vi "Fat A.vi"(11 "GIC Input":T1={"     Use ?\nOff       On"=[FALSE, TRUE, FALSE, TRUE], "Mode:"=FALSE, "Extra Port"="", "Hokuyo Port"="COM7", "Tx Prop  Port"="COM6", "Compass Port"="", "GPS Port"="", "Num of WPs"=0, "WP Lats and Longs"={"WP Lats"=[], "WP Longs"=[]}, "Obst Lats and Longs"={"Obst Lats"=[], "Obst Longs"=[]}, "Parameters"=[], "GPS Data"=[], "Compass"=0.0, "LMS Vector"=[], "Vision Vector"=[], "Direction Cmd"=0.0, "Speed Cmd"=0.0, "WP Vector"=[], "WP Number"=0, "Extra"=0, "SW Map"=[], "Path Cluster"={"Path x node"=[], "Path y node"=[]}, "Sim Course"=[]} {"Obst Lats and Longs"."Obst Longs" format="%#_8g"; "Obst Lats and Longs"."Obst Lats" format="%#_8g"}) -> (3 "GIC Output":T1={"     Use ?\nOff       On"=[FALSE, TRUE, FALSE, TRUE], "Mode:"=FALSE, "Extra Port"="", "Hokuyo Port"="COM7", "Tx Prop  Port"="COM6", "Compass Port"="", "GPS Port"="", "Num of WPs"=0, "WP Lats and Longs"={"WP Lats"=[], "WP Longs"=[]}, "Obst Lats and Longs"={"Obst Lats"=[], "Obst Longs"=[]}, "Parameters"=[], "GPS Data"=[], "Compass"=0.0, "LMS Vector"=[], "Vision Vector"=[], "Direction Cmd"=0.0, "Speed Cmd"=0.0, "WP Vector"=[], "WP Number"=0, "Extra"=0, "SW Map"=[], "Path Cluster"={"Path x node"=[], "Path y node"=[]}, "Sim Course"=[]} {"Obst Lats and Longs"."Obst Longs" format="%#_8g"; "Obst Lats and Longs"."Obst Lats" format="%#_8g"})   [LabVIEW 2014]
panel:
  out "Array":dbl[](array[numeric])
  out "Numeric":dbl
  out "Test SWMap Out":dbl[][](array[numeric])
  in  "Test Fat":dbl=1.0
  # "Fat A"
  # "Input:"
  # "Output:"
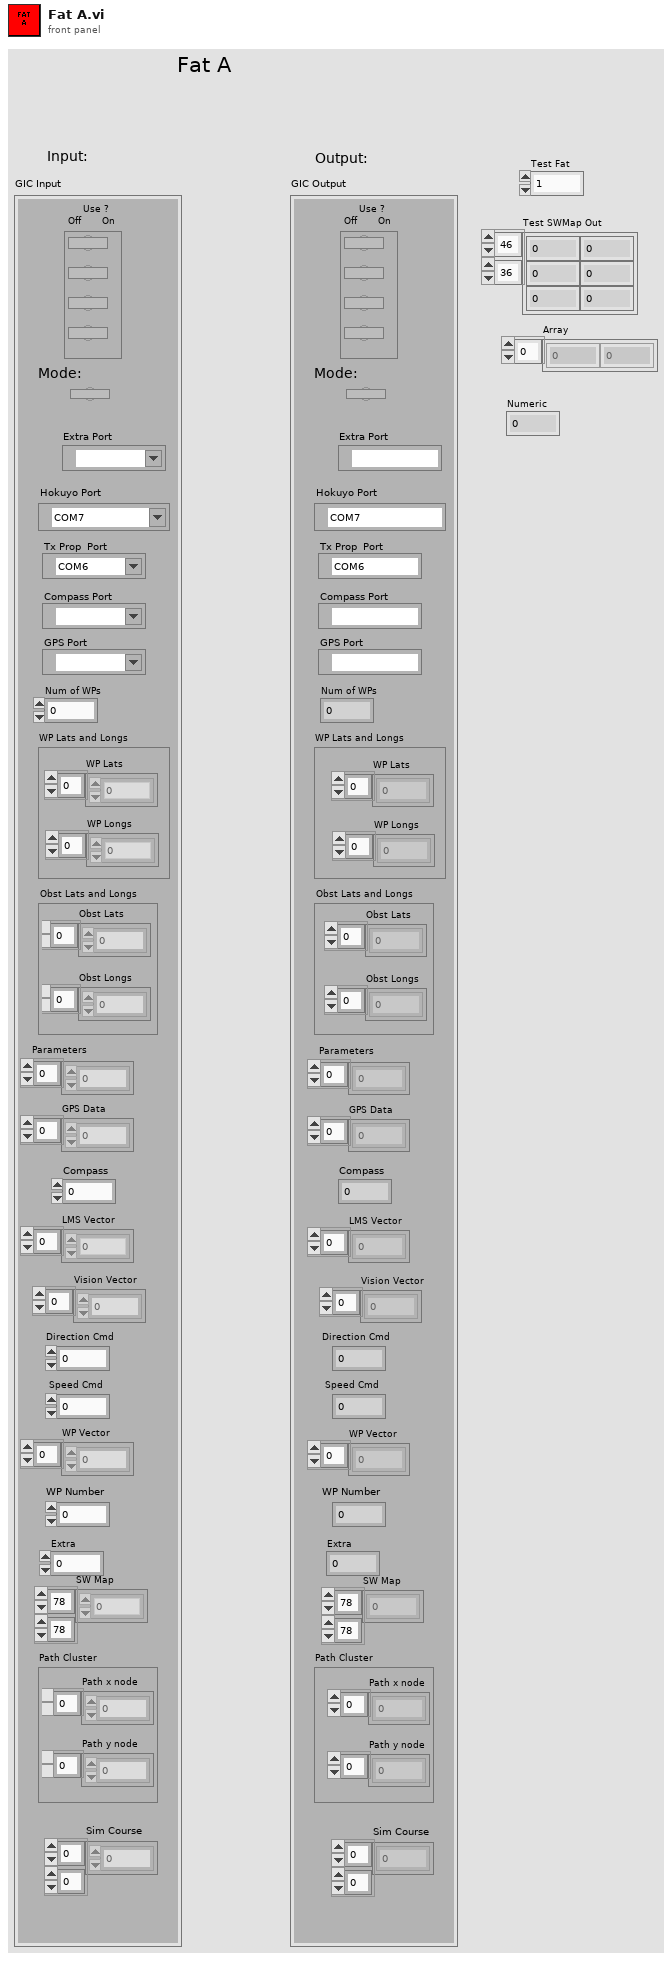
[diagram p1: front panel]
types:
  T1 = cluster{"     Use ?\nOff       On":bool[], "Mode:":bool, "Extra Port":refnum<visa-resource-name>, "Hokuyo Port":refnum<visa-resource-name>, "Tx Prop  Port":refnum<visa-resource-name>, "Compass Port":refnum<visa-resource-name>, "GPS Port":refnum<visa-resource-name>, "Num of WPs":i16, "WP Lats and Longs":cluster{"WP Lats":dbl[], "WP Longs":dbl[]}, "Obst Lats and Longs":cluster{"Obst Lats":dbl[], "Obst Longs":dbl[]}, "Parameters":dbl[], "GPS Data":dbl[], "Compass":dbl, "LMS Vector":dbl[], "Vision Vector":dbl[], "Direction Cmd":dbl, "Speed Cmd":dbl, "WP Vector":dbl[], "WP Number":i32, "Extra":i16, "SW Map":i32[][], "Path Cluster":cluster{"Path x node":dbl[], "Path y node":dbl[]}, "Sim Course":i8[][]}
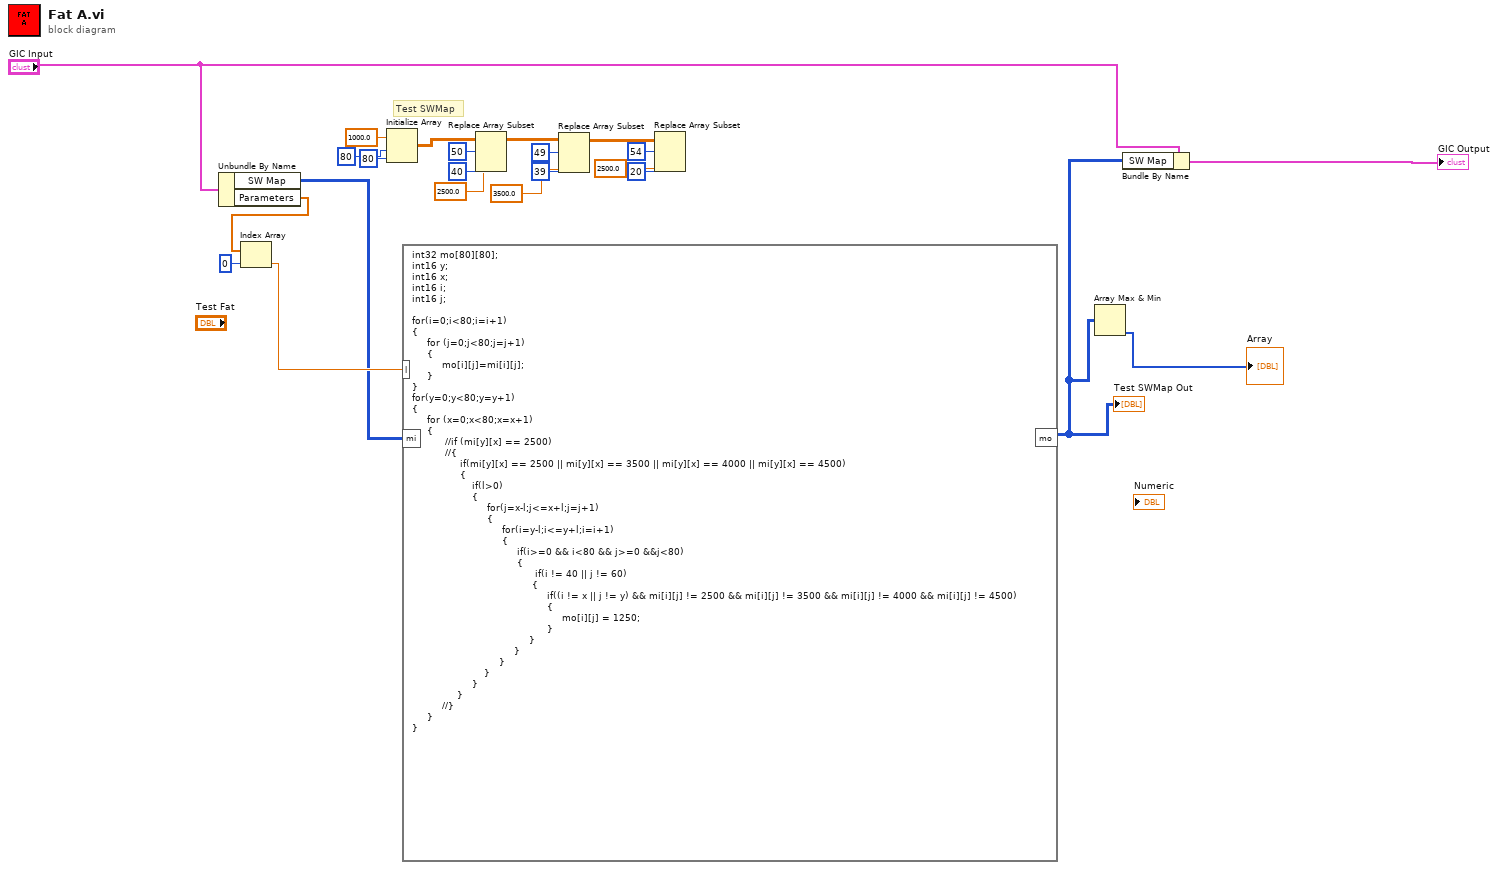
[diagram p0: block diagram]
diagram:
  # "Test SWMap"
  n1 = Unbundle By Name("GIC Input") -> ("SW Map"=w3:i32[][], "Parameters"=w12:dbl[])
  n2 = Index Array(array=w12, index=0) -> (element=w4:dbl)
  n3 = Initialize Array(1000.0 ("element"), 80 ("dimension size"), 80 ("dimension size")) -> (w20:dbl[][])
  n4 = formula code="int32 mo[80][80];\nint16 y;\nint16 x;\nint16 i;\nint16 j;\n\nfor(i=0;i<80;i=i+1)\n{\n     for (j=0;j<80;j=j+1)\n     {\n          mo[i][j]=mi[i][j];\n     }\n}\nfor(y=0;y<80;y=y+1)\n{\n     for (x=0;x<80;x=x+1)\n     {\n           //if (mi[y][x] == 2500)\n           //{\n                if(mi[y][x] == 2500 || mi[y][x] == 3500 || mi[y][x] == 4000 || mi[y][x] == 4500)\n                {\n                    if(l>0)\n                    {\n                         for(j=x-l;j<=x+l;j=j+1)\n                         {\n                              for(i=y-l;i<=y+l;i=i+1)\n                              {\n                                   if(i>=0 && i<80 && j>=0 &&j<80)\n                                   {\n                                         if(i != 40 || j != 60)\n                                        {\n                                             if((i != x || j != y) && mi[i][j] != 2500 && mi[i][j] != 3500 && mi[i][j] != 4000 && mi[i][j] != 4500)\n                                             {\n                                                  mo[i][j] = 1250;\n                                             }\n                                       }\n                                  }\n                             }\n                        }\n                    }\n               } \n          //}\n     }\n}"("mi"=w3, "l"=w4) -> ("mo"=w5:i32[][])
  "Test SWMap Out" <- w5
  n5 = Replace Array Subset(array=w20, new element=2500.0 ("new element/subarray"), index (row)=50, index (col)=40 ("disabled index (col)")) -> (w16:dbl[][])
  n6 = Replace Array Subset(array=w16, new element=3500.0 ("new element/subarray"), index (row)=49, index (col)=39 ("disabled index (col)")) -> (w9:dbl[][])
  n7 = Replace Array Subset(array=w9, new element=2500.0 ("new element/subarray"), index (row)=54, index (col)=20 ("disabled index (col)")) -> ()  [unwired: 1 out]
  n8 = Array Max & Min(array=w5) -> (min index (indices)=→"Array":i32[])  [unwired: 3 out]
  n9 = Bundle By Name(cluster="GIC Input", "SW Map"=w5) -> (→"GIC Output":T1)
